vi "Load New Bitfile.vi"(8 "error in (no error)":errorcluster, 10 "NewVal":path, 11 "Item Ref in":T1 format="%.0x") -> (0 "error out":errorcluster, 3 "Section Ref out":T1 format="%.0x")   [LabVIEW 2015, in "FPGA Addon System Explorer.lvlib"]
uses:
  FPGA Addon System Explorer.lvlib
  <vilib>/NI Veristand/Custom Device API/Custom Device Item Ref.ctl
  Shared/FG Action.ctl
  Shared/Constants.vi
  <vilib>/NI Veristand/Custom Device API/NI VeriStand - Set Item Property.vi
  <vilib>/NI Veristand/Custom Device API/Set Item Property (Variant).vi
  <vilib>/NI Veristand/Custom Device API/NI VeriStand - Get Item Property.vi
  <vilib>/NI Veristand/Custom Device API/Get Item Property (Variant).vi
  <vilib>/NI Veristand/Custom Device Tools/Custom Device Utility Library/NI VeriStand - Search for Item by GUID.vi
  <vilib>/NI Veristand/Custom Device Tools/Custom Device Utility Library/Custom Device Utility Library.lvlib
  Shared/FPGA Addon Shared.lvlib
  <vilib>/NI Veristand/Custom Device API/Custom Device API.lvlib
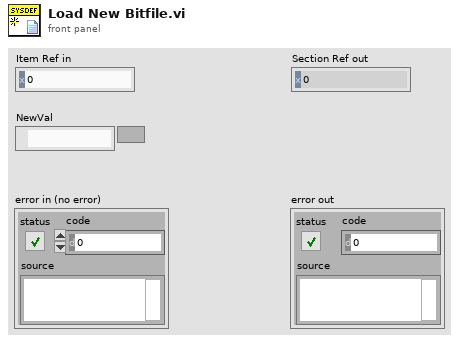
[diagram p1: front panel]
types:
  T1 = typedef "Custom Device API.lvlib/Custom Device Item Ref.ctl" = u64
  T2 = typedef "FPGA Addon Shared.lvlib/FG Action.ctl" = enum8{"GET", "SET"}
  T3 = typedef "Fifo_DMA_Config.ctl" = cluster{"Name":string, "Depth":u32, "Write? (Deprecated:Use Implementation)":bool, "Physical Channel":u32, "Base Address":u32, "Data Width":u32, "Data Type":T4, "FXP Properties":variant, "Write Window Address":u32, "Implementation":T5, "Control Set":u32}
  T4 = typedef "niFpgaDataTypeControl.ctl" = enum32{"Boolean", "I8", "I16", "I32", "I64", "U8", "U16", "U32", "U64", "FXP", "CustomControl", "SGL"}
  T5 = typedef "niFpgaDmaChannelImplementation.ctl" = enum16{"niFpgaTargetToHost", "niFpgaHostToTarget", "niFpgaPeerToPeerWriter", "niFpgaPeerToPeerReader", "niCoreTargetToHost", "niCoreHostToTarget"}
  T6 = typedef "niFpgaBitfileStructure_VI.ctl" = cluster{"Name":string, "RegisterMap":T7[], "Icon":T12}
  T7 = typedef "nirviControlStructure.ctl" = cluster{"Name":string, "Hidden":bool, "Indicator":bool, "Flattened Type":string, "Grouping":cluster{"Grouped":bool, "Member Names":string[], "Member IDs":u32[]}, "Address":u32, "Size":u32, "Class":u32, "Internal":bool, "Typedef":T8, "ID":u32, "Bidirectional":bool, "Synchronous":bool, "Mechanical Action":T9, "Sub Controls":T10[], "Access May Timeout":bool, "Register Node":bool}
  T8 = typedef "nirviTypdefDescription.ctl" = cluster{"Typedef":bool, "Path":path}
  T9 = typedef "nirviMechanicalAction.ctl" = enum8{"Switch When Pressed", "Switch When Released", "Switch Until Released", "Latch When Pressed", "Latch When Released", "Latch Until Released"}
  T10 = typedef "nirviSubControlStructure.ctl" = cluster{"Name":string, "flattened Type":string, "Cluster Information":T11, "Typedef":T8}
  T11 = typedef "nirviClusterElementControl.ctl" = cluster{"Name Hierarchy":string[], "Item Order":u32[]}
  T12 = typedef "imagedata.ctl" = cluster{"image type":i32, "image depth":i32, "image":u8[], "mask":u8[], "colors":u32[], "Rectangle":cluster{"left":i16, "top":i16, "right":i16, "bottom":i16}}
  T13 = typedef "FPGA Addon Shared.lvlib/Register Information.ctl" = cluster{"Name":string, "Data Type":T14, "Default Value":variant}
  T14 = typedef "FPGA Addon Shared.lvlib/Data Type.ctl" = enum8{"<Null>", "I8", "I16", "I32", "I64", "U8", "U16", "U32", "U64", "SGL", "Boolean", "Analog PWM In Settings", "Analog PWM In", "Digital PWM In Settings", "Digital PWM In", "Digital PWM Out", "Sine Out", "FXP+/-24.5", "FXP+/-16.5", "FXP+/-32.8", "FXP+/-64.32", "FXP+/-16.7"}
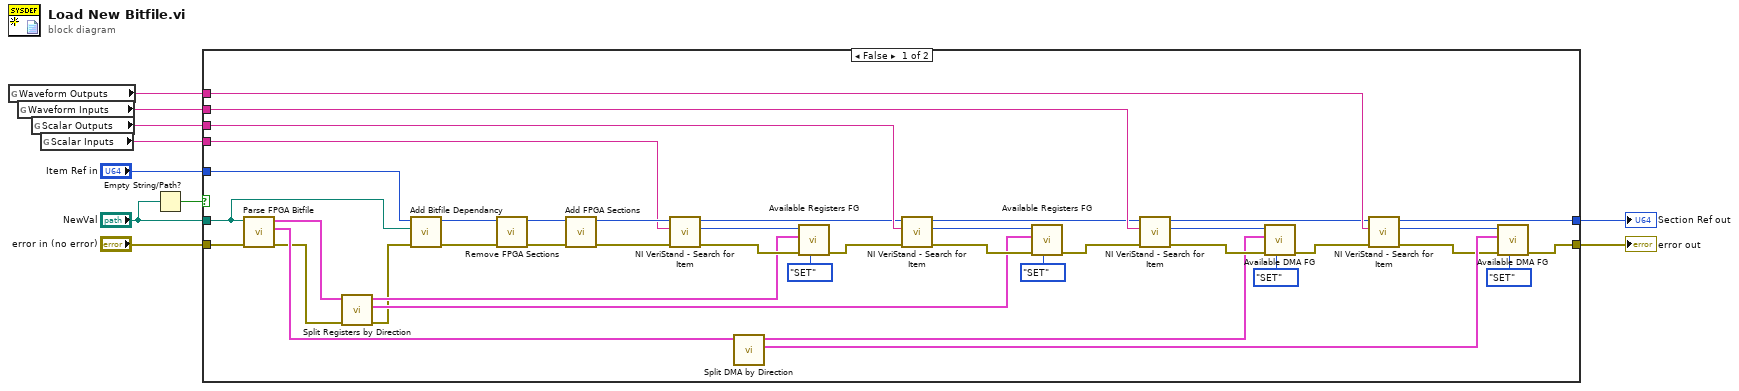
[diagram p0: block diagram]
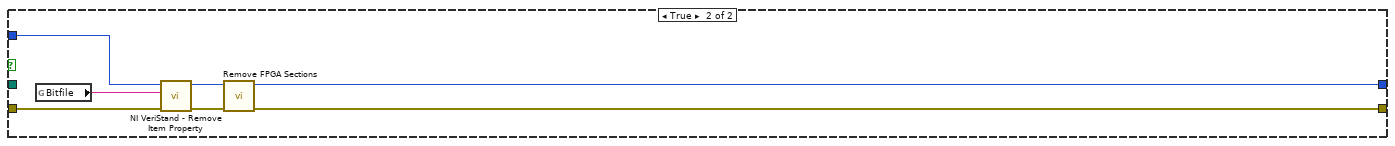
[diagram p2: hidden frame]
diagram:
  n1 = global read "Constants.vi" "Waveform Outputs"() -> (w7:string)
  n2 = global read "Constants.vi" "Waveform Inputs"() -> (w8:string)
  n3 = global read "Constants.vi" "Scalar Outputs"() -> (w9:string)
  n4 = global read "Constants.vi" "Scalar Inputs"() -> (w10:string)
  n5 = Empty String/Path?(string/path="NewVal") -> (empty?=w4:bool)
  n6 = case shown="False" w4 {
    tunnel: "NewVal" -> [w17 _]
    tunnel: "error in (no error)" -> [w51 w53]
    tunnel: w10 -> [w46 _]
    tunnel: w9 -> [w43 _]
    tunnel: w8 -> [w39 _]
    tunnel: w7 -> [w38 _]
    tunnel: [w23 w58] -> w6
    tunnel: [w21 w57] -> w5
    tunnel: "Item Ref in" -> [w16 w55]
    frame False {
      n7 = call "Parse FPGA Bitfile.vi"("error in (no error)"=w51, "Path"=w17) -> ("error out"=w12:errorcluster, "DMA configuration array"=w45:T3[], "vi info"=w44:T6)  [unwired: 7 in]
      n8 = call "Split Registers by Direction.vi"("error in"=w12, "vi info"=w44) -> ("error out"=w11:errorcluster, "Controls"=w13:T13[], "Indicator"=w14:T13[])  [unwired: 7 in]
      n9 = call "Add Bitfile Dependancy.vi"("error in (no error)"=w11, "Path"=w17, "Item Ref in"=w16) -> ("error out"=w18:errorcluster, "Item Ref out"=w15:T1)  [unwired: 7 in]
      n10 = call "Remove FPGA Sections.vi"("error in (no error)"=w18, "Item Ref in"=w15) -> ("error out"=w19:errorcluster, "Item Ref out"=w20:T1)  [unwired: 8 in]
      n11 = call "Add FPGA Sections.vi"("error in (no error)"=w19, "Node Ptr"=w20) -> ("error out"=w49:errorcluster, "Parent Ref out"=w50:T1)  [unwired: 8 in]
      n12 = call-poly <vilib>:"NI VeriStand - Search for Item.vi"("error in"=w49, "Item GUID"=w46, "Section Ref in"=w50) -> ("error out"=w48:errorcluster, "Item Ref"=w47:T1, "Section Ref out"=w41:T1)  [unwired: 5 in, 1 out]
      n13 = call "Split DMA by Direction.vi"("DMA configuration array"=w45) -> ("HostToTarget"=w25:T3[], "TargetToHost"=w30:T3[])  [unwired: 9 in]
      n14 = call "Available Registers FG.vi"("Action"=FG_Action."SET", "error in (no error)"=w48, "Available Registers"=w14, "Item Ref"=w47) -> ("error out"=w42:errorcluster)  [unwired: 5 in, 2 out]
      n15 = call-poly <vilib>:"NI VeriStand - Search for Item.vi"("error in"=w42, "Item GUID"=w43, "Section Ref in"=w41) -> ("error out"=w34:errorcluster, "Item Ref"=w33:T1, "Section Ref out"=w37:T1)  [unwired: 5 in, 1 out]
      n16 = call "Available Registers FG.vi"("Action"=FG_Action."SET", "error in (no error)"=w34, "Available Registers"=w13, "Item Ref"=w33) -> ("error out"=w32:errorcluster)  [unwired: 5 in, 2 out]
      n17 = call-poly <vilib>:"NI VeriStand - Search for Item.vi"("error in"=w32, "Item GUID"=w39, "Section Ref in"=w37) -> ("error out"=w31:errorcluster, "Item Ref"=w40:T1, "Section Ref out"=w27:T1)  [unwired: 5 in, 1 out]
      n18 = call "Available DMA FG.vi"("Action"=FG_Action."SET", "error in (no error)"=w31, "Available DMA"=w30, "Item Ref"=w40) -> ("error out"=w28:errorcluster)  [unwired: 5 in, 2 out]
      n19 = call-poly <vilib>:"NI VeriStand - Search for Item.vi"("error in"=w28, "Item GUID"=w38, "Section Ref in"=w27) -> ("error out"=w24:errorcluster, "Item Ref"=w26:T1, "Section Ref out"=w21:T1)  [unwired: 5 in, 1 out]
      n20 = call "Available DMA FG.vi"("Action"=FG_Action."SET", "error in (no error)"=w24, "Available DMA"=w25, "Item Ref"=w26) -> ("error out"=w23:errorcluster)  [unwired: 5 in, 2 out]
    }
    frame True {
      n21 = global read "Constants.vi" "Bitfile"() -> (w56:string)
      n22 = call <vilib>:"NI VeriStand - Remove Item Property.vi"("error in (no error)"=w53, "Property Name"=w56, "Item Ref in"=w55) -> ("error out"=w52:errorcluster, "Item Ref out"=w54:T1)  [unwired: 6 in, 1 out]
      n23 = call "Remove FPGA Sections.vi"("error in (no error)"=w52, "Item Ref in"=w54) -> ("error out"=w58:errorcluster, "Item Ref out"=w57:T1)  [unwired: 8 in]
    }
  }
  "error out" <- w6
  "Section Ref out" <- w5
